vi "buscarCCD.vi"(10 "Orden":T1(array[ring])=[enum."espejos", enum."voltaje", enum."polarizador", enum."potenciometro ", enum."CCD"]) -> (1 "Orden 2":T1(array[ring]), 2 "ccd?":bool)   [LabVIEW 2016]
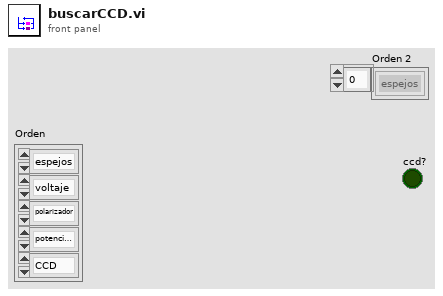
[diagram p1: front panel]
types:
  T1 = enum16{"espejos", "polarizador", "voltaje", "potenciometro ", "CCD", "lockin", "laser", "ninguno"}[]
  T2 = enum16{"espejos", "polarizador", "voltaje", "potenciometro ", "CCD", "lockin", "laser", "ninguno"}
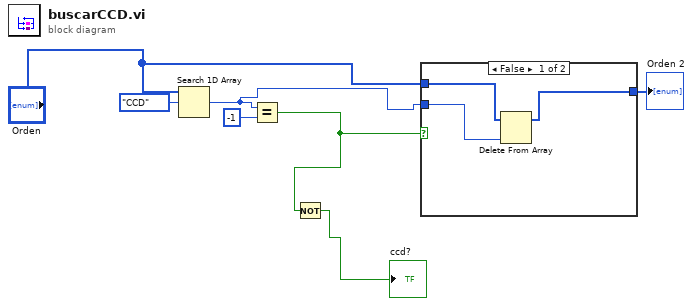
[diagram p0: block diagram]
diagram:
  n1 = Search 1D Array(1D array="Orden", element=T2."CCD") -> (index of element=w3:i32)  [unwired: 1 in]
  n2 = Equal?(x=w3, y=-1) -> (x = y?=w2:bool)
  n3 = Not(x=w2) -> (.not. x?=→"ccd?":bool)
  n4 = case shown="False" w2 {
    tunnel: [w8 w11] -> w4
    tunnel: "Orden" -> [w10 w11]
    tunnel: w3 -> [w9 _]
    frame False {
      n5 = Delete From Array(array=w10, index=w9) -> (array with subset deleted=w8:T1)  [unwired: 1 in, 1 out]
    }
    frame True {
    }
  }
  "Orden 2" <- w4
